vi "correccionColor.vi"() -> ()   [LabVIEW 2020]
panel:
  in  "Nombre Grafica":string
  in  "Nombre imagen":string
  in  "Save Button":bool
  out "Histograma original":dbl[][](graph)
  out "Histograma modificado":dbl[][](graph)
  in  "P":dbl(slide) scale=0.255..255.0
  in  "c":dbl(slide) scale=1.0..255.0
  out "XY Graph":cluster{i32[], dbl[]}(graph)
  in  "Enum":T1(ring)
  out "new picture":picture
  in  "path to JPEG file":path=path "C:/Users/dtrej/Downloads/SVA 06 HISTOGRAMA-20250430T011009Z-001/SVA 06 HISTOGRAMA/1.jpg"
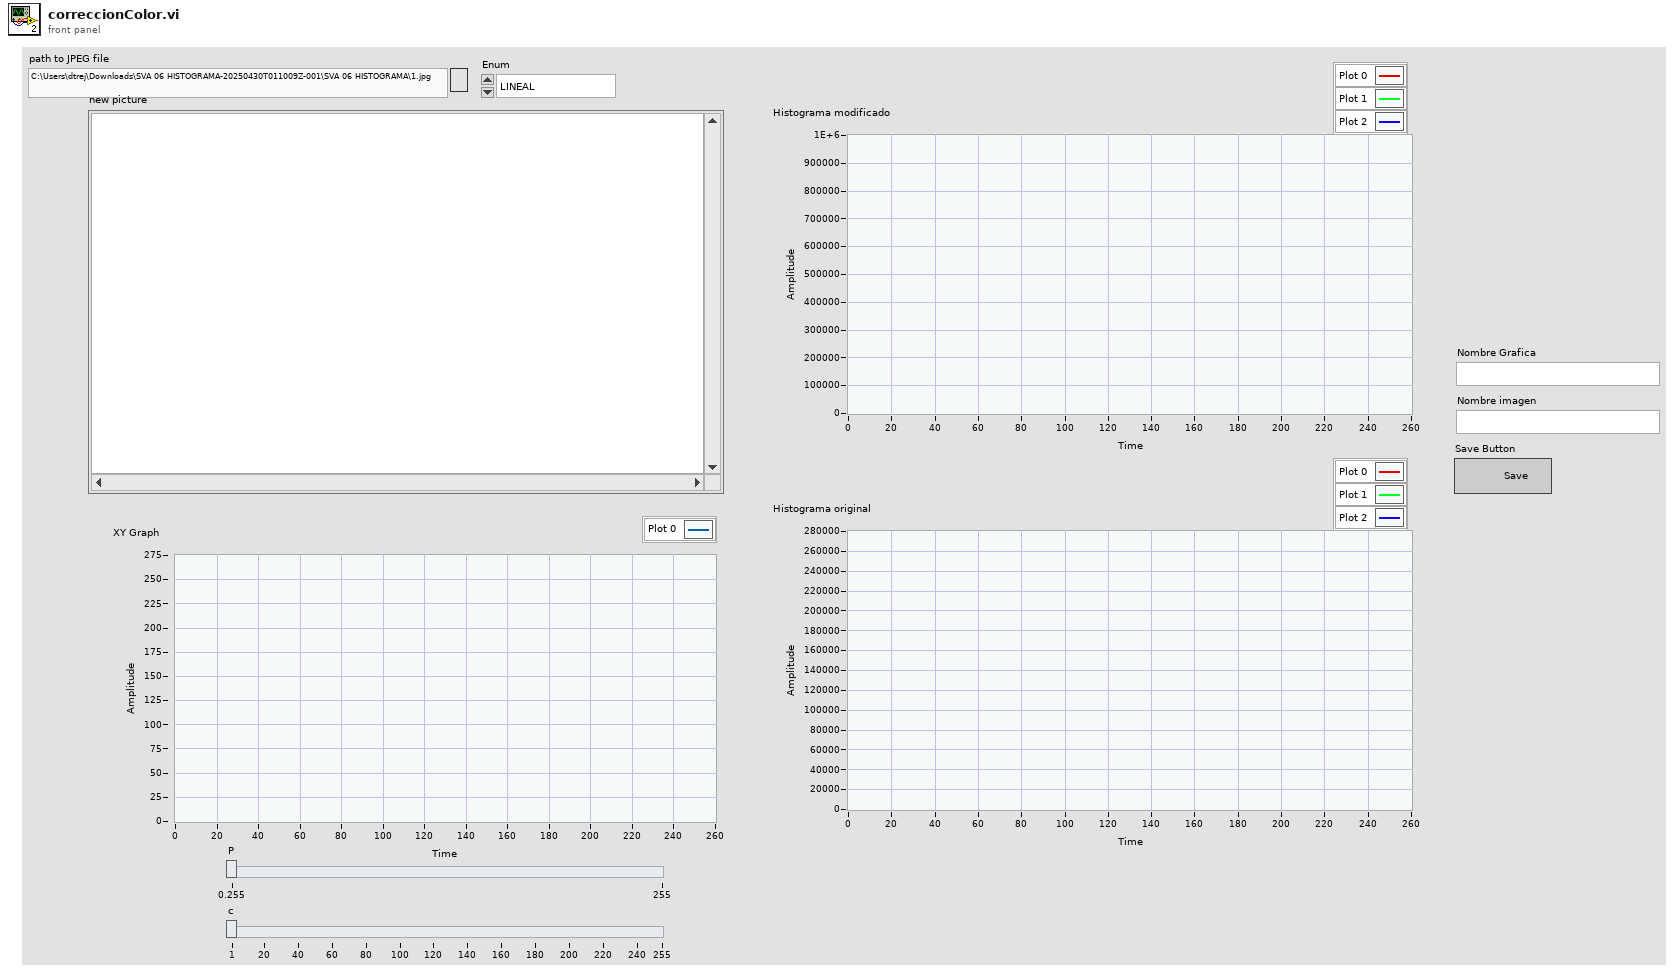
[diagram p1: front panel]
types:
  T1 = enum16{"LINEAL", "CUADRATICO", "RAIZ", "LOGARITMICO", "EXPONENCIAL", "POTENCIA", "POTENCIA INVERSA", "GUSSIANA"}
  T2 = typedef "imagedata.ctl" = cluster{"image type":i32, "image depth":i32, "image":u8[], "mask":u8[], "colors":u32[], "Rectangle":cluster{"left":i16, "top":i16, "right":i16, "bottom":i16}}
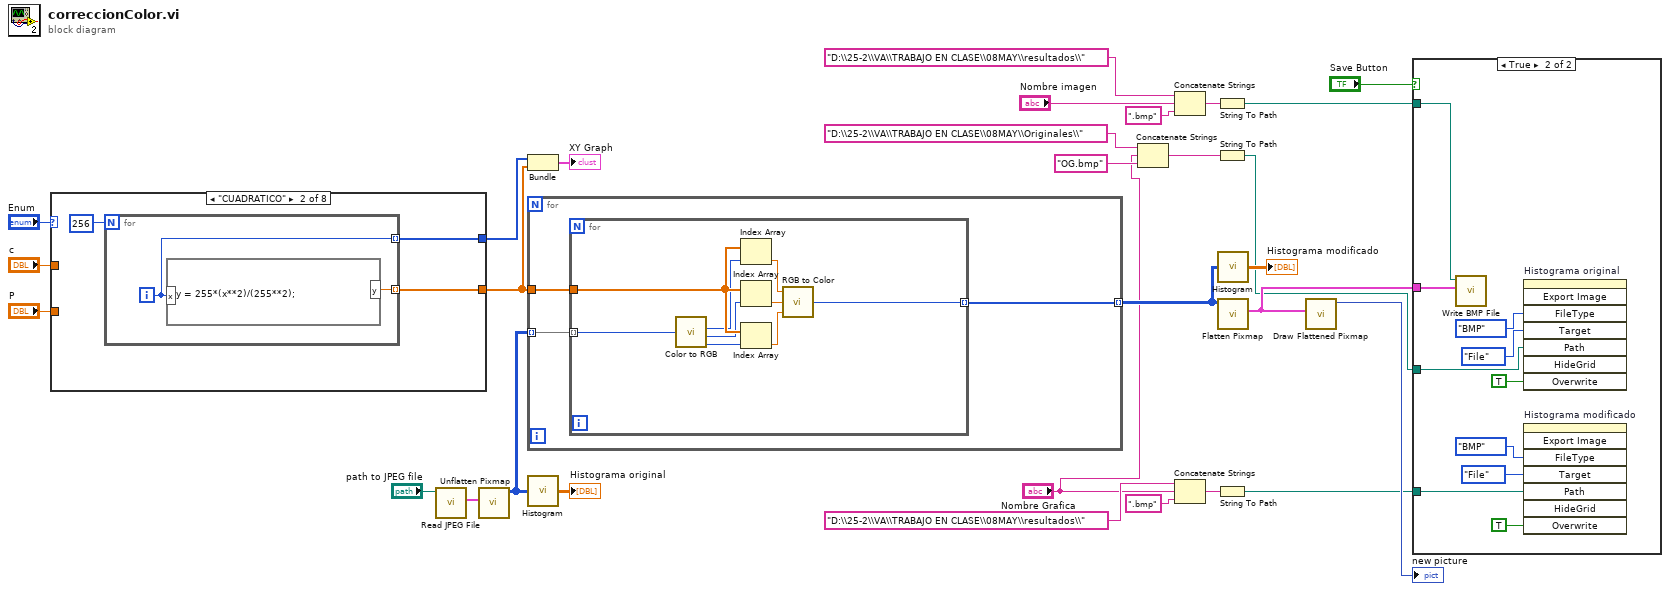
[diagram p0: block diagram]
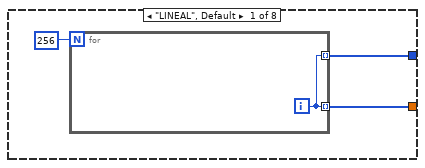
[diagram p3: hidden frame]
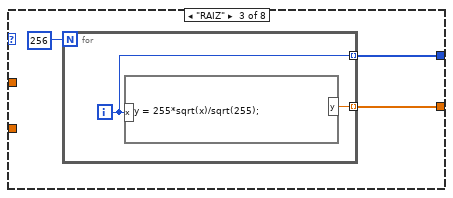
[diagram p4: hidden frame]
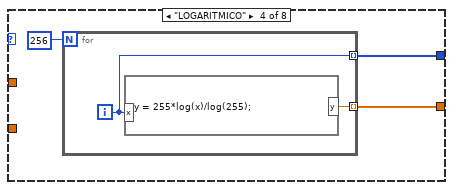
[diagram p5: hidden frame]
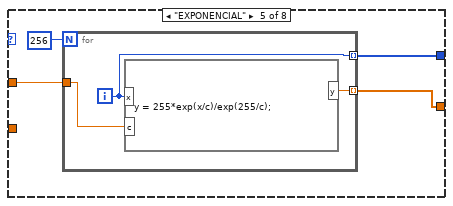
[diagram p6: hidden frame]
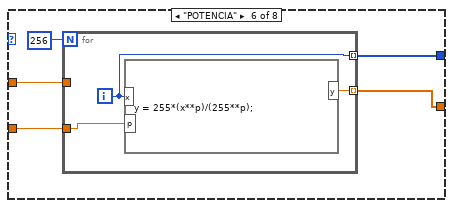
[diagram p7: hidden frame]
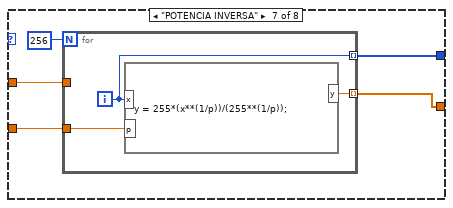
[diagram p8: hidden frame]
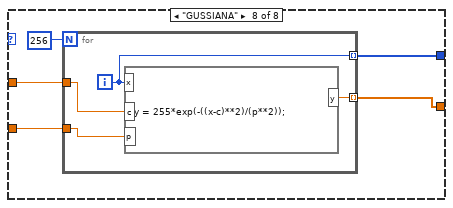
[diagram p9: hidden frame]
diagram:
  n1 = case shown="\"CUADRATICO\"" "Enum" {
    tunnel: [w31 w34 w39 w44 w50 w58 w66 w74] -> w23
    tunnel: [w30 w35 w40 w45 w51 w59 w67 w75] -> w25
    tunnel: "c" -> [_ _ _ _ w49 w57 w65 w73]
    tunnel: "P" -> [_ _ _ _ _ w56 w64 w72]
    frame "LINEAL", Default {
      n2 = for {
        N: 256 -> [_]
        tunnel: [w33] -> w30 mode=indexing
        tunnel: [w33] -> w31 mode=indexing
        i -> [w33]
      }
    }
    frame "CUADRATICO" {
      n3 = for {
        N: 256 -> [_]
        tunnel: [w37] -> w35 mode=indexing
        tunnel: [w38] -> w34 mode=indexing
        i -> [w37]
        n4 = formula code="y = 255*(x**2)/(255**2);"("x"=w37) -> ("y"=w38:dbl)
      }
    }
    frame "RAIZ" {
      n5 = for {
        N: 256 -> [_]
        tunnel: [w42] -> w40 mode=indexing
        tunnel: [w43] -> w39 mode=indexing
        i -> [w42]
        n6 = formula code="y = 255*sqrt(x)/sqrt(255);"("x"=w42) -> ("y"=w43:dbl)
      }
    }
    frame "LOGARITMICO" {
      n7 = for {
        N: 256 -> [_]
        tunnel: [w47] -> w45 mode=indexing
        tunnel: [w48] -> w44 mode=indexing
        i -> [w47]
        n8 = formula code="y = 255*log(x)/log(255);"("x"=w47) -> ("y"=w48:dbl)
      }
    }
    frame "EXPONENCIAL" {
      n9 = for {
        N: 256 -> [_]
        tunnel: [w54] -> w51 mode=indexing
        tunnel: [w55] -> w50 mode=indexing
        tunnel: w49 -> [w53]
        i -> [w54]
        n10 = formula code="y = 255*exp(x/c)/exp(255/c);"("x"=w54, "c"=w53) -> ("y"=w55:dbl)
      }
    }
    frame "POTENCIA" {
      n11 = for {
        N: 256 -> [_]
        tunnel: [w62] -> w59 mode=indexing
        tunnel: [w63] -> w58 mode=indexing
        tunnel: w57 -> [_]
        tunnel: w56 -> [w61]
        i -> [w62]
        n12 = formula code="y = 255*(x**p)/(255**p);"("x"=w62, "p"=w61) -> ("y"=w63:dbl)
      }
    }
    frame "POTENCIA INVERSA" {
      n13 = for {
        N: 256 -> [_]
        tunnel: [w70] -> w67 mode=indexing
        tunnel: [w71] -> w66 mode=indexing
        tunnel: w65 -> [_]
        tunnel: w64 -> [w69]
        i -> [w70]
        n14 = formula code="y = 255*(x**(1/p))/(255**(1/p));"("x"=w70, "p"=w69) -> ("y"=w71:dbl)
      }
    }
    frame "GUSSIANA" {
      n15 = for {
        N: 256 -> [_]
        tunnel: [w79] -> w75 mode=indexing
        tunnel: [w80] -> w74 mode=indexing
        tunnel: w73 -> [w77]
        tunnel: w72 -> [w78]
        i -> [w79]
        n16 = formula code="y = 255*exp(-((x-c)**2)/(p**2));"("x"=w79, "p"=w78, "c"=w77) -> ("y"=w80:dbl)
      }
    }
  }
  n17 = call <vilib>:"Read JPEG File.vi"("path to JPEG file"="path to JPEG file") -> ("image data"=w27:T2)  [unwired: 8 in, 2 out]
  n18 = call <vilib>:"Unflatten Pixmap.vi"("image data"=w27) -> ("24-bit pixmap"=w17:u32[][])  [unwired: 4 in, 6 out]
  n19 = Bundle(w25, w23) -> (→"XY Graph":cluster{i32[], dbl[]})  [unwired: 1 in]
  n20 = for {
    tunnel: w17 -> [w83] mode=indexing
    tunnel: [w82] -> w19 mode=indexing
    tunnel: w23 -> [w81]
    n21 = for {
      tunnel: w83 -> [w92] mode=indexing
      tunnel: [w91] -> w82 mode=indexing
      tunnel: w81 -> [w90]
      n22 = call <vilib>:"Color to RGB.vi"("Color"=w92) -> ("R"=w89:u8, "G"=w88:u8, "B"=w87:u8)  [unwired: 1 out]
      n23 = Index Array(array=w90, index=w89) -> (element=w84:dbl)
      n24 = Index Array(array=w90, index=w88) -> (element=w85:dbl)
      n25 = Index Array(array=w90, index=w87) -> (element=w86:dbl)
      n26 = call <vilib>:"RGB to Color.vi"("B"=w86, "G"=w85, "R"=w84) -> ("Color"=w91:u32)
    }
  }
  n27 = call "Histogram.vi"("Array in"=w17) -> ("Array out"=→"Histograma original":dbl[][])
  n28 = Concatenate Strings("D:\\25-2\\VA\\TRABAJO EN CLASE\\08MAY\\Originales\\", "Nombre Grafica", "OG.bmp") -> (w3:string)
  n29 = Concatenate Strings("D:\\25-2\\VA\\TRABAJO EN CLASE\\08MAY\\resultados\\", "Nombre imagen", ".bmp") -> (w11:string)
  n30 = Concatenate Strings("D:\\25-2\\VA\\TRABAJO EN CLASE\\08MAY\\resultados\\", "Nombre Grafica", ".bmp") -> (w9:string)
  n31 = String To Path(string=w11) -> (path=w10:path)
  n32 = String To Path(string=w3) -> (path=w2:path)
  n33 = String To Path(string=w9) -> (path=w6:path)
  n34 = call "Histogram.vi"("Array in"=w19) -> ("Array out"=→"Histograma modificado":dbl[][])
  n35 = call <vilib>:"Flatten Pixmap.vi"("24-bit pixmap"=w19) -> ("image data"=w16:T2)  [unwired: 10 in]
  n36 = call <vilib>:"Draw Flattened Pixmap.vi"("image data"=w16) -> ("new picture"=→"new picture":picture)  [unwired: 8 in]
  n37 = case shown="True" "Save Button" {
    tunnel: w16 -> [_ w102]
    tunnel: w10 -> [_ w99]
    tunnel: w6 -> [_ w98]
    tunnel: w2 -> [_ w93]
    frame False {
    }
    frame True {
      n38 = call <vilib>:"Write BMP File.vi"("image data"=w102, "path to BMP file"=w99) -> ()  [unwired: 8 in, 2 out]
      n39 = invoke on="Histograma original" class="WFGraph (strict)" method="Export Image"("FileType"=enum32{"BMP", "EPS", "EMF", "PICT"}."BMP" ("File Type"), "Target"=enum32{"File", "Clipboard"}."File", "Path"=w93, "Overwrite"=TRUE ("Always Overwrite")) -> ()  [unwired: 4 in, 8 out]
      n40 = invoke on="Histograma modificado" class="WFGraph (strict)" method="Export Image"("FileType"=enum32{"BMP", "EPS", "EMF", "PICT"}."BMP" ("File Type"), "Target"=enum32{"File", "Clipboard"}."File", "Path"=w98, "Overwrite"=TRUE ("Always Overwrite")) -> ()  [unwired: 4 in, 8 out]
    }
  }
